vi "Show.vi"(6 "Force? (true)":bool=TRUE, 7 "Subpanel Ref (empty: open detached)":refnum<vi>, 8 "error in (no error)":errorcluster, 11 "SMO.UI_Embed In":refnum<class "SMO.UI_Embed.lvclass">) -> (0 "error out":errorcluster, 3 "SMO.UI_Embed Out":refnum<class "SMO.UI_Embed.lvclass">)   [LabVIEW 2019, in "SMO.UI_Embed.lvclass"]
doc: "Opens the front panel of the SMO.UI_Embed either as a standalone VI or embedded in a subpanel. If the Force? input is set to TRUE, this method will force the VI to be subpanelled or to be open stand-alone, based on the Subpanel Ref input."
uses:
  SMO.UI_Embed.lvclass
  Typedefs/SMO.UI_Embed State--enum.ctl
panel:
  # "For instructions on how to use the JKI State Machine Objects, examples and video tutorials, visit:\nhttp://jki.net/state-machine-objects/\n\nJKI State Machine Objects™\nhttp://jki.net/state-machine-objects/\nCopyright (C) 2005-2015, JKI <info@jki.net>\nALL RIGHTS RESERVED"
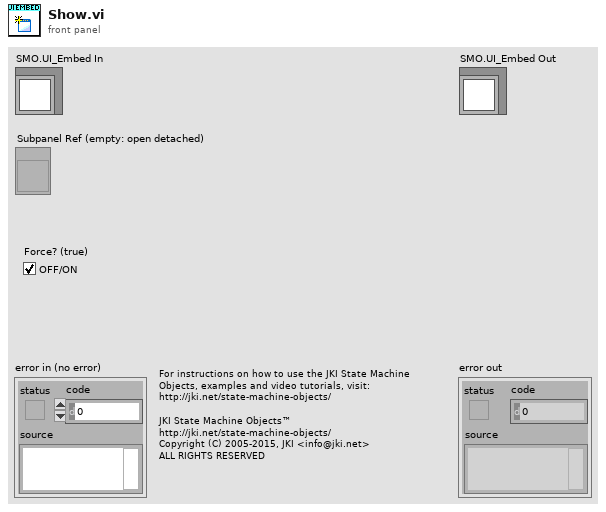
[diagram p1: front panel]
types:
  T1 = typedef "SMO.UI_Embed.lvclass/SMO.UI_Embed State--enum.ctl" = enum16{"unknown", "Opened", "Embedded", "Closed"}
  T2 = enum32{"Invalid", "Standard", "Closed", "Hidden", "Minimized", "Maximized"}
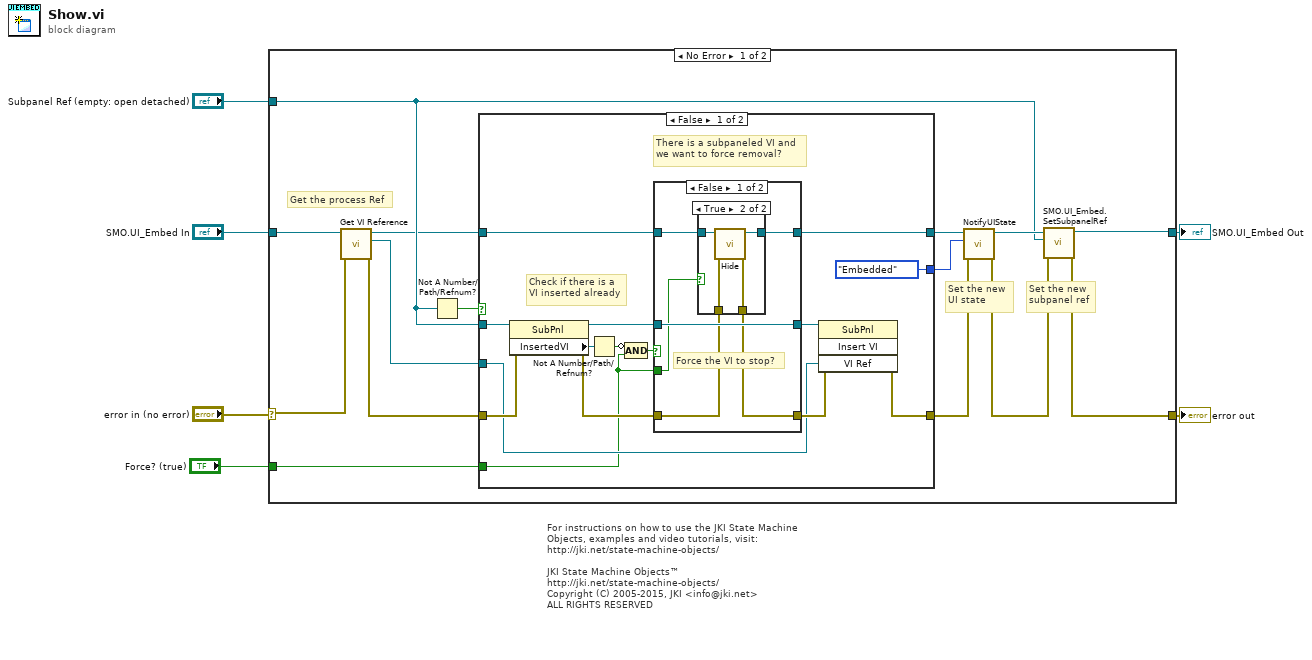
[diagram p0: block diagram]
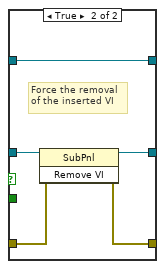
[diagram p3: hidden frame]
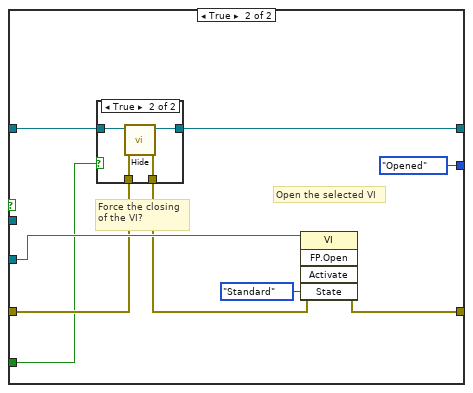
[diagram p4: hidden frame]
diagram:
  # "For instructions on how to use the JKI State Machine Objects, examples and video tutorials, visit:\nhttp://jki.net/state-machine-objects/\n\nJKI State Machine Objects™\nhttp://jki.net/state-machine-objects/\nCopyright (C) 2005-2015, JKI <info@jki.net>\nALL RIGHTS RESERVED"
  n1 = case shown="No Error" "error in (no error)" {
    selector: "error in (no error)" -> [w9 w70]
    tunnel: "SMO.UI_Embed In" -> [w11 w69]
    tunnel: [w13 w70] -> w5
    tunnel: [w15 w69] -> w4
    tunnel: "Subpanel Ref (empty: open detached)" -> [w12 _]
    tunnel: "Force? (true)" -> [w18 _]
    frame No Error {
      # "Set the new \nUI state"
      # "Set the new \nsubpanel ref"
      # "Get the process Ref"
      n2 = call-dynamic "Get VI Reference.vi"("error in (no error)"=w9, "SMO.UI_Embed In"=w11) -> ("error out"=w8:errorcluster, "VI Reference"=w7:refnum<vi>, "SMO.UI_Embed Out"=w10:refnum<class "SMO.UI_Embed.lvclass">)  [unwired: 7 in]
      n3 = Not A Number/Path/Refnum?(number/path/refnum=w12) -> (NaN/Path/Refnum?=w21:bool)
      n4 = case shown="False" w21 {
        tunnel: w7 -> [w23 w62]
        tunnel: w8 -> [w33 w56]
        tunnel: [w36 w60] -> w20
        tunnel: w12 -> [w34 _]
        tunnel: [SMO.UI_Embed_State--enum."Embedded" ("UI State") SMO.UI_Embed_State--enum."Opened" ("UI State")] -> w19
        tunnel: w18 -> [w22 w54]
        tunnel: [w25 w57] -> w17
        tunnel: w10 -> [w24 w58]
        frame False {
          # "There is a subpaneled VI and\nwe want to force removal?"
          # "Check if there is a \nVI inserted already"
          n5 = property class="SubPnl"(reference=w34, error in=w33) -> (reference out=w29:refnum<vi>, error out=w28:errorcluster, "InsertedVI"=w26:refnum<vi>)
          n6 = Not A Number/Path/Refnum?(number/path/refnum=w26) -> (NaN/Path/Refnum?=w32:bool)
          n7 = Compound Arithmetic op=AND(invert w32, w22) -> (w31:bool)
          n8 = case shown="False" w31 {
            tunnel: [w42 w52] -> w30
            tunnel: w29 -> [w42 w53]
            tunnel: w28 -> [w39 w51]
            tunnel: [w38 w50] -> w27
            tunnel: [w40 w49] -> w25
            tunnel: w24 -> [w41 w49]
            tunnel: w22 -> [w37 _]
            frame False {
              # "Force the VI to stop?"
              n9 = case shown="True" w37 {
                tunnel: w41 -> [w44 w48]
                tunnel: [w44 w47] -> w40
                tunnel: w39 -> [w43 w46]
                tunnel: [w43 w45] -> w38
                frame False {
                }
                frame True {
                  n10 = call "Hide.vi"("error in (no error)"=w46, "SMO.UI_Embed In"=w48) -> ("error out"=w45:errorcluster, "SMO.UI_Embed Out"=w47:refnum<class "SMO.UI_Embed.lvclass">)  [unwired: 8 in]
                }
              }
            }
            frame True {
              # "Force the removal\nof the inserted VI"
              n11 = invoke on="Invoke Node" class="SubPnl" method="Remove VI"(reference=w53, error in=w51) -> (reference out=w52:refnum<vi>, error out=w50:errorcluster)  [unwired: 1 in, 1 out]
            }
          }
          n12 = invoke on="Invoke Node" class="SubPnl" method="Insert VI"(reference=w30, error in=w27, "VI Ref"=w23) -> (error out=w36:errorcluster)  [unwired: 1 in, 3 out]
        }
        frame True {
          # "Force the closing\nof the VI?"
          # "Open the selected VI"
          n13 = case shown="True" w54 {
            tunnel: w58 -> [w64 w68]
            tunnel: [w64 w67] -> w57
            tunnel: w56 -> [w63 w66]
            tunnel: [w63 w65] -> w55
            frame False {
            }
            frame True {
              n14 = call "Hide.vi"("error in (no error)"=w66, "SMO.UI_Embed In"=w68) -> ("error out"=w65:errorcluster, "SMO.UI_Embed Out"=w67:refnum<class "SMO.UI_Embed.lvclass">)  [unwired: 8 in]
            }
          }
          n15 = invoke class="VI" method="FP.Open"(reference=w62, error in=w55, "State"=T2."Standard") -> (error out=w60:errorcluster)  [unwired: 2 in, 4 out]
        }
      }
      n16 = call "NotifyUIState.vi"("error in (no error)"=w20, "UI State"=w19, "SMO.UI_Embed In"=w17) -> ("error out"=w14:errorcluster, "SMO.UI_Embed Out"=w16:refnum<class "SMO.UI_Embed.lvclass">)  [unwired: 7 in]
      n17 = call "SMO.UI_Embed.SetSubpanelRef.vi"("error in (no error)"=w14, "Subpanel Ref"=w12, "SMO.UI_Embed"=w16) -> ("error out"=w13:errorcluster, "SMO.UI_Embed out"=w15:refnum<class "SMO.UI_Embed.lvclass">)  [unwired: 7 in]
    }
    frame Error {
    }
  }
  "error out" <- w5
  "SMO.UI_Embed Out" <- w4
